vi "ATF-Button logic.vi"(7 "option":T8, 8 "error in":errorcluster, 11 "?":T2) -> (0 "error out":errorcluster, 3 "Data out":T1(array[ring]))   [LabVIEW 2022 SP3]
uses:
  Controls/ATF-button logic.ctl
  Controls/main case.ctl
  Controls/SeCrTs-boolean ref.ctl
  Controls/SeCrTs-EPV .ctl
  Controls/Commands to log.ctl
  UI Message handler/Message Queue/All Message Queues.ctl
  UI Message handler/Message Queue/Message Cluster.ctl
  Controls/SeCrTs-Notifier ctl.ctl
  Controls/SeCrTs-NS Data type.ctl
  a8c6863f-0f0f-4e96-9570-dcb746d39beb.vi
  UI Message handler/Message Queue/Message Queue.lvlib
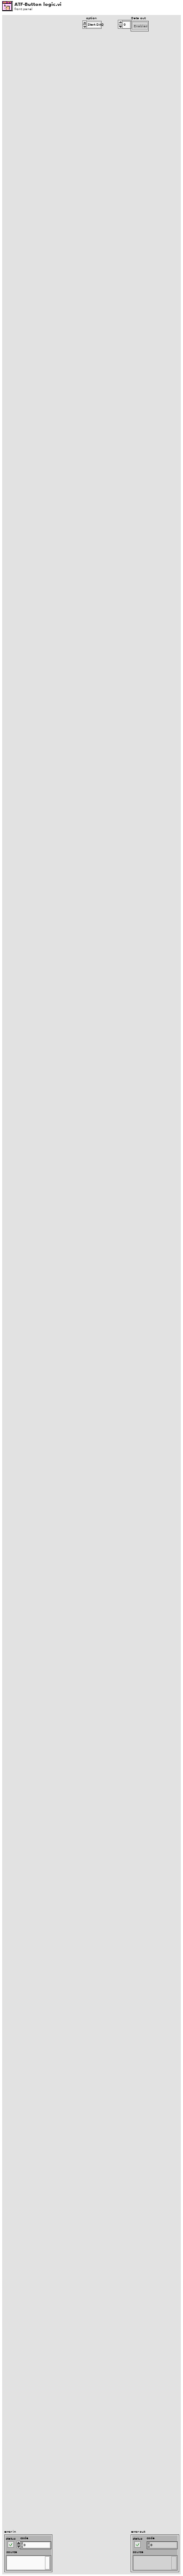
[diagram p1: front panel]
types:
  T1 = enum8{"Enabled", "Disabled", "Disabled and Grayed Out"}[]
  T2 = typedef "main case.ctl" = cluster{"Bol":T3, "EPV":T4, "Covers":cluster{"cover":refnum<vi>, "Login screen cover":refnum<vi>, "cover Motor":refnum<vi>}, "Log cmd":T5, "STORAGE IP":string, "PUMP IP":string, "Storage con":bool, "Pumb con":bool, "que ref":T6, "not ref":T7, "notification":cluster{"C/NC":bool, "Start/Stop Log":bool[], "Log Name":string, "Config":cluster{"AO config":cluster{"Channel_Name":string, "Channel_Number":string, "Default_Value":dbl, "Units":string}[], "AI config":cluster{"Channel_Name":string, "Channel_Number":string, "Pre_Scale_min":dbl, "Pre_Scale_max":dbl, "Sensor_min":dbl, "Sensor_max":dbl, "Units":string}[], "DI config":cluster{"Channel_Name":string, "Channel_Number":string, "Default_Value":bool, "DI invert?":bool}[], "DO config":cluster{"Channel_Name":string, "Channel_Number":string, "Default_Value":bool, "DO invert?":bool}[], "TC config":cluster{"Channel_Name":string, "Channel_Number":string, "Pre_Scale_min":dbl, "Pre_Scale_max":dbl, "units":i32, " type":i32}[], "ACC config":cluster{"Channel_Name":string, "Channel_Number":string, "Pre_Scale_min":dbl, "Pre_Scale_max":dbl, "Terminal configuration":i32, "Sensitivity":dbl, "Sensitivity units":i32}[], "SG config":cluster{"Channel_Name":string, "Channel_Number":string, "Pre_Scale_min":dbl, "Pre_Scale_max":dbl}[], "Strain Gauge Settings":cluster{"poisson ratio":dbl, "nominal gage resistance":dbl, "gage factor":dbl}, "Bridge Settings":cluster{"voltage excitation value":dbl, "voltage excitation source":i32, "initial bridge voltage":dbl, "lead wire resistance":dbl, "strain configuration":i32}, "Sample Rate":cluster{"AI Sample Rate":dbl[], "AO Sample Rate":dbl[], "DI Sample Rate":dbl[], "TC Sample Rate":dbl[], "DO Sample Rate":dbl[], "SG Sample Rate":dbl[], "ACC Sample Rate":dbl[]}, "Drive":cluster{"Drive_Health":bool, "Drive_Frequency":u32, "Drive_Status":bool, "Drive_RPM":u32, "Drive_Direction":bool, "Acceleration state":bool, "Steady state":bool, "Deceleration state":bool, "Drive_Enable":bool, "Drive set_RPM":dbl}}, "Log min":dbl}}
  T3 = typedef "SeCrTs-boolean ref.ctl" = cluster{"Connect RT":refnum<vi>, "START DAQ":refnum<vi>, "STOP DAQ":refnum<vi>, "DAQ SETTING":refnum<vi>, "START LOG":refnum<vi>, "STOP LOG":refnum<vi>, "Connect Drive ATF":refnum<vi>, "Update drive ATF":refnum<vi>, "Gate driver ATF":refnum<vi>, "Motor On ATF":refnum<vi>, "ADC reset ATF":refnum<vi>, "Gate driver ATF 2":refnum<vi>, "Motor off ATF":refnum<vi>, "MCU reset ATF":refnum<vi>, "Connect Drive Lox":refnum<vi>, "Update drive lox":refnum<vi>, "Gate driver- LOX":refnum<vi>, "Motor On lox":refnum<vi>, "Adc reset lox":refnum<vi>, "MCU Reset -LOX":refnum<vi>, "Motor Off lox":refnum<vi>, "Connect ppsu":refnum<vi>, "update ppsu":refnum<vi>, "DC on":refnum<vi>, "Alarm ack":refnum<vi>, "DC off":refnum<vi>, "Ms initialize":refnum<vi>, "Exit RT":refnum<vi>, "ABORT":refnum<vi>, "HOLD UPDATE":refnum<vi>, "Log type":refnum<vi>, "PUMP IP":refnum<vi>, "STORAGE IP":refnum<vi>}
  T4 = typedef "SeCrTs-EPV .ctl" = cluster{"F_EPV_131":refnum<vi>, "F_EPV_132":refnum<vi>, "F_EPV_136":refnum<vi>, "F_EPV_21":refnum<vi>, "F_EPV_41":refnum<vi>, "N_EPV_68":refnum<vi>, "N_EPV_ 69":refnum<vi>, "N_EPV_ 33":refnum<vi>, "F_EPV_142":refnum<vi>, "F_EPV_28":refnum<vi>, "N_EPV_203":refnum<vi>, "N_EPV_206":refnum<vi>, "F_EPV_75":refnum<vi>, "C_EPV_2":refnum<vi>, "C_EPV_7":refnum<vi>, "C_EPV_8":refnum<vi>, "C_EPV_123":refnum<vi>, "C_EPV_124":refnum<vi>, "C_EPV_127":refnum<vi>, "N_EPV_62a":refnum<vi>, "N_EPV_62b":refnum<vi>, "N_EPV_61":refnum<vi>, "G_EPV_51":refnum<vi>, "N_EPV_141":refnum<vi>, "C_EPV_803":refnum<vi>, "C_EPV_18":refnum<vi>, "C_EPV_1352":refnum<vi>, "N_EPV_202":refnum<vi>, "C_EPV_16":refnum<vi>}
  T5 = typedef "Commands to log.ctl" = cluster{"C/NC":bool, "Start/Stop Log":bool[], "Log Name":string, "Config":cluster{"AO config":cluster{"Channel_Name":string, "Channel_Number":string, "Default_Value":dbl, "Units":string}[], "AI config":cluster{"Channel_Name":string, "Channel_Number":string, "Pre_Scale_min":dbl, "Pre_Scale_max":dbl, "Sensor_min":dbl, "Sensor_max":dbl, "Units":string}[], "DI config":cluster{"Channel_Name":string, "Channel_Number":string, "Default_Value":bool, "DI invert?":bool}[], "DO config":cluster{"Channel_Name":string, "Channel_Number":string, "Default_Value":bool, "DO invert?":bool}[], "TC config":cluster{"Channel_Name":string, "Channel_Number":string, "Pre_Scale_min":dbl, "Pre_Scale_max":dbl, "units":i32, " type":i32}[], "ACC config":cluster{"Channel_Name":string, "Channel_Number":string, "Pre_Scale_min":dbl, "Pre_Scale_max":dbl, "Terminal configuration":i32, "Sensitivity":dbl, "Sensitivity units":i32}[], "SG config":cluster{"Channel_Name":string, "Channel_Number":string, "Pre_Scale_min":dbl, "Pre_Scale_max":dbl}[], "Strain Gauge Settings":cluster{"poisson ratio":dbl, "nominal gage resistance":dbl, "gage factor":dbl}, "Bridge Settings":cluster{"voltage excitation value":dbl, "voltage excitation source":i32, "initial bridge voltage":dbl, "lead wire resistance":dbl, "strain configuration":i32}, "Sample Rate":cluster{"AI Sample Rate":dbl[], "AO Sample Rate":dbl[], "DI Sample Rate":dbl[], "TC Sample Rate":dbl[], "DO Sample Rate":dbl[], "SG Sample Rate":dbl[], "ACC Sample Rate":dbl[]}}, "Log min":dbl, "Drive":cluster{"Drive_Health":bool, "Drive_Frequency":u32, "Drive_Status":bool, "Drive_RPM":u32, "Drive_Direction":bool, "Acceleration state":bool, "Steady state":bool, "Deceleration state":bool, "Drive_Enable":bool, "Drive set_RPM":dbl}, "HOLD UPDATE":bool}
  T6 = typedef "Message Queue.lvlib/All Message Queues.ctl" = cluster{"UI":refnum<queue>, "ER":refnum<queue>, "Ev":refnum<queue>, "R ER Storage":refnum<queue>, "PPSU":refnum<queue>, "R ER Pumb":refnum<queue>}
  T7 = typedef "SeCrTs-Notifier ctl.ctl" = cluster{"Storage Data":refnum<notifier>, "Pumb Data":refnum<notifier>, "Log cmd":refnum<notifier>}
  T8 = typedef "ATF-button logic.ctl" = enum16{"Start DAQ", "Stop DAQ", "Start Datalog", "Stop Log", "Hold Update", "Connect RT", "Disconnect RT", "Enable IP", "Disable IP", "init", "Connect drive", "Update drive", "Motor on", "Motor off", "Exit drive", "Connect PPSU", "Update PPSU", "DC on", "DC off"}
  T9 = cluster{"ref":refnum<vi>[], "state":enum8{"Enabled", "Disabled", "Disabled and Grayed Out"}[]}
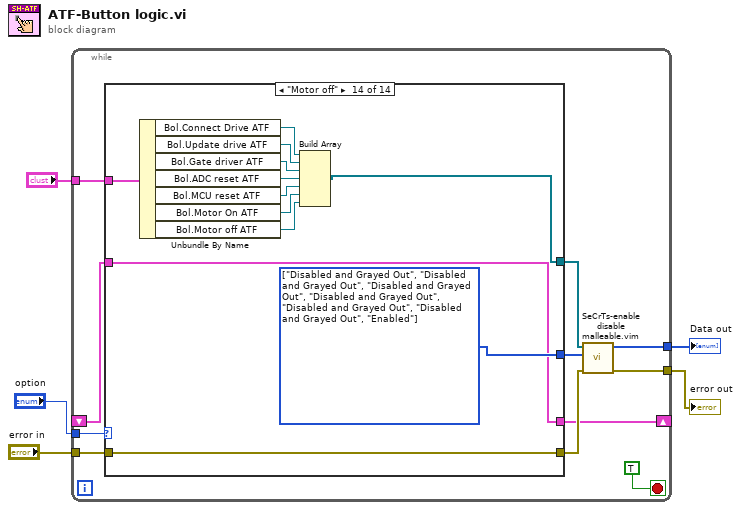
[diagram p0: block diagram]
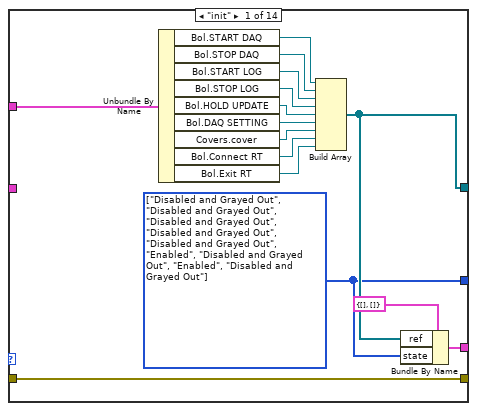
[diagram p2: hidden frame]
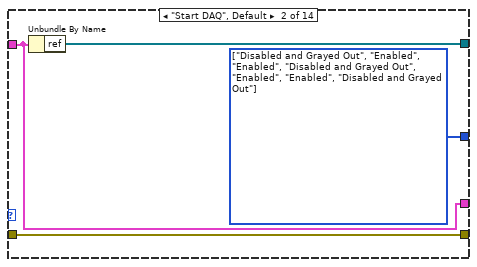
[diagram p3: hidden frame]
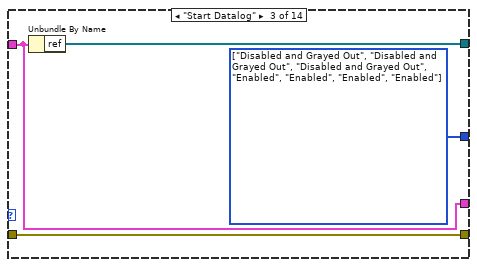
[diagram p4: hidden frame]
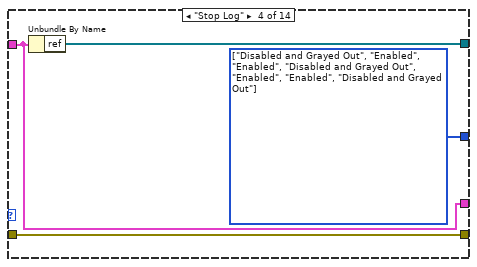
[diagram p5: hidden frame]
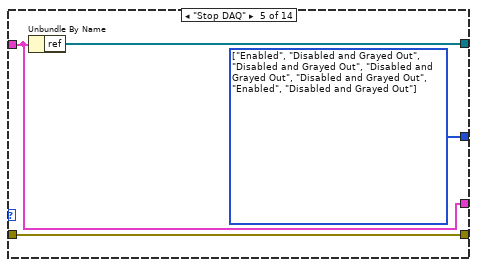
[diagram p6: hidden frame]
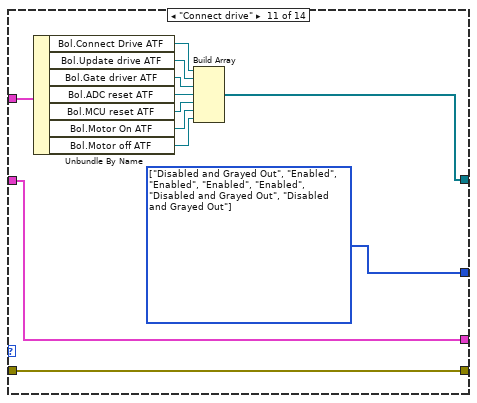
[diagram p12: hidden frame]
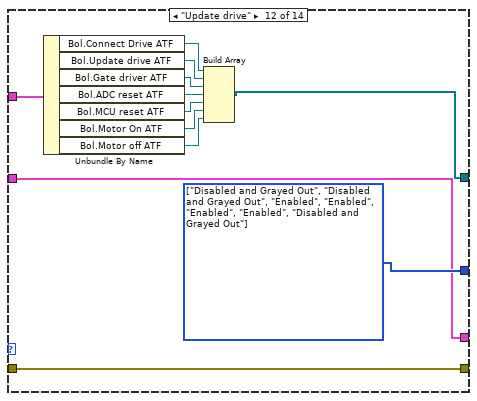
[diagram p13: hidden frame]
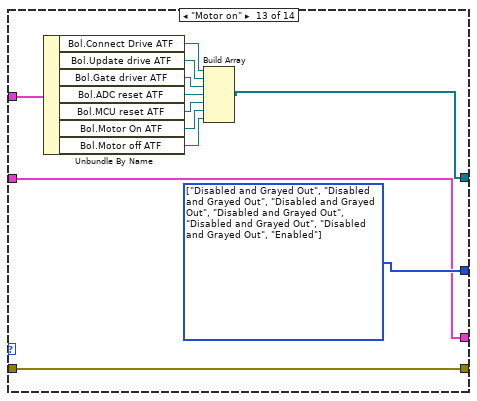
[diagram p14: hidden frame]
diagram:
  n1 = while {
    tunnel: "error in" -> [w15]
    tunnel: [w13] -> w4
    tunnel: "option" -> [w12]
    shift-right: [w10] -> _
    shift-left: _ -> [w11]
    tunnel: [w7] -> w2
    tunnel: "?" -> [w6]
    stop <- TRUE stop-if-true
    n2 = case shown="\"Motor off\"" w12 {
      tunnel: w15 -> [w31 w35 w39 w43 w47 w49 w51 w53 w55 w57 w69 w81 w93 w105]
      tunnel: [w31 w35 w39 w43 w47 w49 w51 w53 w55 w57 w69 w81 w93 w105] -> w14
      tunnel: w11 -> [_ w33 w37 w40 w45 w48 w50 w52 w54 w56 w58 w79 w91 w103]
      tunnel: [w23 w33 w37 w40 w45 w48 w50 w52 w54 w56 w58 w79 w91 w103] -> w10
      tunnel: [w22 w34 w38 w42 w46 _ _ _ _ _ w60 w70 w82 w94] -> w9
      tunnel: [w21 w32 w36 w41 w44 _ _ _ _ _ w59 w80 w92 w104] -> w8
      tunnel: w6 -> [w17 _ _ _ _ _ _ _ _ _ w68 w71 w83 w95]
      frame "init" {
        w21 = T1 [enum."Disabled and Grayed Out", enum."Disabled and Grayed Out", enum."Disabled and Grayed Out", enum."Disabled and Grayed Out", enum."Disabled and Grayed Out", enum."Enabled", enum."Disabled and Grayed Out", enum."Enabled", enum."Disabled and Grayed Out"] items=["Enabled", "Disabled", "Disabled and Grayed Out"] ("Disabled")
        n3 = Unbundle By Name(w17) -> ("Bol.START DAQ"=w30:refnum<vi>, "Bol.STOP DAQ"=w29:refnum<vi>, "Bol.START LOG"=w28:refnum<vi>, "Bol.STOP LOG"=w27:refnum<vi>, "Bol.HOLD UPDATE"=w26:refnum<vi>, "Bol.DAQ SETTING"=w25:refnum<vi>, "Covers.cover"=w24:refnum<vi>, "Bol.Connect RT"=w20:refnum<vi>, "Bol.Exit RT"=w18:refnum<vi>)
        n4 = Build Array(w30, w29, w28, w27, w26, w25, w24, w20, w18) -> (w22:refnum<vi>[])
        n5 = Bundle By Name(cluster=T9 {"ref"=[], "state"=[]}, "ref"=w22, "state"=w21) -> (w23:T9)
      }
      frame "Start DAQ", Default {
        w32 = T1 [enum."Disabled and Grayed Out", enum."Enabled", enum."Enabled", enum."Disabled and Grayed Out", enum."Enabled", enum."Enabled", enum."Disabled and Grayed Out"] items=["Enabled", "Disabled", "Disabled and Grayed Out"] ("Disabled")
        n6 = Unbundle By Name(w33) -> ("ref"=w34:refnum<vi>[])
      }
      frame "Start Datalog" {
        w36 = T1 [enum."Disabled and Grayed Out", enum."Disabled and Grayed Out", enum."Disabled and Grayed Out", enum."Enabled", enum."Enabled", enum."Enabled", enum."Enabled"] items=["Enabled", "Disabled", "Disabled and Grayed Out"] ("Disabled")
        n7 = Unbundle By Name(w37) -> ("ref"=w38:refnum<vi>[])
      }
      frame "Stop Log" {
        w41 = T1 [enum."Disabled and Grayed Out", enum."Enabled", enum."Enabled", enum."Disabled and Grayed Out", enum."Enabled", enum."Enabled", enum."Disabled and Grayed Out"] items=["Enabled", "Disabled", "Disabled and Grayed Out"] ("Disabled")
        n8 = Unbundle By Name(w40) -> ("ref"=w42:refnum<vi>[])
      }
      frame "Stop DAQ" {
        w44 = T1 [enum."Enabled", enum."Disabled and Grayed Out", enum."Disabled and Grayed Out", enum."Disabled and Grayed Out", enum."Disabled and Grayed Out", enum."Enabled", enum."Disabled and Grayed Out"] items=["Enabled", "Disabled", "Disabled and Grayed Out"] ("Disabled")
        n9 = Unbundle By Name(w45) -> ("ref"=w46:refnum<vi>[])
      }
      frame "Hold Update" {
      }
      frame "Connect RT" {
      }
      frame "Disconnect RT" {
      }
      frame "Enable IP" {
      }
      frame "Disable IP" {
      }
      frame "Connect drive" {
        w59 = T1 [enum."Disabled and Grayed Out", enum."Enabled", enum."Enabled", enum."Enabled", enum."Enabled", enum."Disabled and Grayed Out", enum."Disabled and Grayed Out"] items=["Enabled", "Disabled", "Disabled and Grayed Out"] ("Disabled")
        n10 = Unbundle By Name(w68) -> ("Bol.Connect Drive ATF"=w67:refnum<vi>, "Bol.Update drive ATF"=w66:refnum<vi>, "Bol.Gate driver ATF"=w65:refnum<vi>, "Bol.ADC reset ATF"=w64:refnum<vi>, "Bol.MCU reset ATF"=w63:refnum<vi>, "Bol.Motor On ATF"=w62:refnum<vi>, "Bol.Motor off ATF"=w61:refnum<vi>)
        n11 = Build Array(w67, w66, w65, w64, w63, w62, w61) -> (w60:refnum<vi>[])
      }
      frame "Update drive" {
        w80 = T1 [enum."Disabled and Grayed Out", enum."Disabled and Grayed Out", enum."Enabled", enum."Enabled", enum."Enabled", enum."Enabled", enum."Disabled and Grayed Out"] items=["Enabled", "Disabled", "Disabled and Grayed Out"] ("Disabled")
        n12 = Unbundle By Name(w71) -> ("Bol.Connect Drive ATF"=w78:refnum<vi>, "Bol.Update drive ATF"=w77:refnum<vi>, "Bol.Gate driver ATF"=w76:refnum<vi>, "Bol.ADC reset ATF"=w75:refnum<vi>, "Bol.MCU reset ATF"=w74:refnum<vi>, "Bol.Motor On ATF"=w73:refnum<vi>, "Bol.Motor off ATF"=w72:refnum<vi>)
        n13 = Build Array(w78, w77, w76, w75, w74, w73, w72) -> (w70:refnum<vi>[])
      }
      frame "Motor on" {
        w92 = T1 [enum."Disabled and Grayed Out", enum."Disabled and Grayed Out", enum."Disabled and Grayed Out", enum."Disabled and Grayed Out", enum."Disabled and Grayed Out", enum."Disabled and Grayed Out", enum."Enabled"] items=["Enabled", "Disabled", "Disabled and Grayed Out"] ("Disabled")
        n14 = Unbundle By Name(w83) -> ("Bol.Connect Drive ATF"=w90:refnum<vi>, "Bol.Update drive ATF"=w89:refnum<vi>, "Bol.Gate driver ATF"=w88:refnum<vi>, "Bol.ADC reset ATF"=w87:refnum<vi>, "Bol.MCU reset ATF"=w86:refnum<vi>, "Bol.Motor On ATF"=w85:refnum<vi>, "Bol.Motor off ATF"=w84:refnum<vi>)
        n15 = Build Array(w90, w89, w88, w87, w86, w85, w84) -> (w82:refnum<vi>[])
      }
      frame "Motor off" {
        w104 = T1 [enum."Disabled and Grayed Out", enum."Disabled and Grayed Out", enum."Disabled and Grayed Out", enum."Disabled and Grayed Out", enum."Disabled and Grayed Out", enum."Disabled and Grayed Out", enum."Enabled"] items=["Enabled", "Disabled", "Disabled and Grayed Out"] ("Disabled")
        n16 = Unbundle By Name(w95) -> ("Bol.Connect Drive ATF"=w102:refnum<vi>, "Bol.Update drive ATF"=w101:refnum<vi>, "Bol.Gate driver ATF"=w100:refnum<vi>, "Bol.ADC reset ATF"=w99:refnum<vi>, "Bol.MCU reset ATF"=w98:refnum<vi>, "Bol.Motor On ATF"=w97:refnum<vi>, "Bol.Motor off ATF"=w96:refnum<vi>)
        n17 = Build Array(w102, w101, w100, w99, w98, w97, w96) -> (w94:refnum<vi>[])
      }
    }
    n18 = call "SeCrTs-enable disable malleable.vim"("error in"=w14, "Data"=w8, "Ref in"=w9) -> ("error out"=w13:errorcluster, "Data out"=w7:T1)  [unwired: 7 in]
  }
  "error out" <- w4
  "Data out" <- w2
